vi "Simple Vector Field Histogram.vi"(7 "panic range":T1, 8 "error in (no error)":errorcluster, 9 "distance threshold":dbl, 10 "direction angles":dbl[](array[numeric]), 11 "distances":dbl[](array[numeric])) -> (0 "error out":errorcluster, 1 "histogram":cluster{"Direction":dbl[], dbl[]}[](graph)=[{"Direction"=array[277 elements], [0.5, 0.5, 0.5, 0.5, 0.5, 0.5, 0.5, 0.5, 0.5, 0.5, 0.5, 0.5, 0.5, 0.5, 0.5, 0.5, 0.5, 0.5, 0.5, 0.5, 0.5, 0.5, 0.5, 0.5, 0.5, 0.5, 0.5, 0.5, 0.5, 0.5, 0.5, 0.5, 0.5, 0.5, 0.5, 0.5, 0.5, 0.5, 0.5, 0.5, 0.5, 0.5, 0.5, 0.5, 0.5, 0.5, 0.5, 0.5, 0.5, 0.5, 0.5, 0.5, 0.5, 0.5, 0.5, 0.5, 0.5, 0.5, 0.5, 0.5, 0.5, 0.5, 0.5, 0.5, 0.5, 0.5, 0.5, 0.5, 0.5, 0.5, 0.5, 0.5, 0.5, 0.5, 0.5, 0.5, 0.5, 0.5, 0.5, 0.5, 0.5, 0.5, 0.5, 0.5, 0.5, 0.5, 0.5, 0.5, 0.5, 0.5, 0.5, 0.5, 0.5, 0.5, 0.5, 0.5, 0.5, 0.5, 0.5, 0.5, 0.5, 0.5, 0.5, 0.5, 0.5, 0.5, 0.5, 0.5, 0.5, 0.5, 0.5, 0.5, 0.5, 0.5, 0.5, 0.5, 0.5, 0.5, 0.5, 0.5, 0.5, 0.5, 0.5, 0.5, 0.5, 0.5, 0.5, 0.5, 0.5, 0.5, 0.5, 0.5, 0.5, 0.5, 0.5, 0.5, 0.5, 0.5, 0.5, 0.5, 0.5, 0.5, 0.5, 0.5, 0.5, 0.5, 0.5, 0.5, 0.5, 0.5, 0.5, 0.5, 0.5, 0.5, 0.5, 0.5, 0.5, 0.5, 0.5, 0.5, 0.5, 0.5, 0.5, 0.5, 0.5, 0.5, 0.5, 0.5, 0.5, 0.5, 0.5, 0.5, 0.5, 0.5, 0.5, 0.5, 0.5, 0.5, 0.5, 0.5, 0.5, 0.5, 0.5, 0.5, 0.5, 0.5, 0.5, 0.5, 0.5, 0.5, 0.5, 0.5, 0.5, 0.5, 0.5, 0.5, 0.5, 0.5, 0.5, 0.5, 0.5, 0.5, 0.5, 0.5, 0.5, 0.5, 0.5, 0.5, 0.5, 0.5, 0.5, 0.5, 0.5, 0.5, 0.5, 0.5, 0.5, 0.5, 0.5, 0.5, 0.5, 0.5, 0.5, 0.5, 0.5, 0.5, 0.5, 0.5, 0.5, 0.5, 0.5, 0.5, 0.5, 0.5, 0.5, 0.5, 0.5, 0.5, 0.5, 0.5, 0.5, 0.5, 0.5, 0.5, 0.5, 0.5, 0.5, 0.5, 0.5, 0.5, 0.5, 0.5, 0.5, 0.5, 0.5, 0.5, 0.5, 0.5, 0.5, 0.5, 0.5, 0.5, 0.5, 0.5, 0.5, 0.5, 0.5, 0.5, 0.5, 0.5, 0.5, 0.5, 0.5, 0.5, 0.5, 0.5, 0.5]}, {"Direction"=array[683 elements], [0.0, 1.0, 1.0, 1.0, 1.0, 1.0, 1.0, 1.0, 1.0, 1.0, 1.0, 1.0, 1.0, 1.0, 1.0, 1.0, 1.0, 1.0, 1.0, 1.0, 1.0, 1.0, 1.0, 1.0, 1.0, 1.0, 1.0, 1.0, 1.0, 1.0, 1.0, 1.0, 1.0, 1.0, 1.0, 1.0, 1.0, 1.0, 1.0, 1.0, 1.0, 1.0, 1.0, 1.0, 1.0, 1.0, 1.0, 1.0, 1.0, 1.0, 1.0, 1.0, 1.0, 1.0, 1.0, 1.0, 1.0, 1.0, 1.0, 1.0, 1.0, 1.0, 1.0, 1.0, 1.0, 1.0, 1.0, 1.0, 1.0, 1.0, 1.0, 1.0, 1.0, 1.0, 1.0, 1.0, 1.0, 1.0, 1.0, 1.0, 1.0, 1.0, 1.0, 1.0, 1.0, 1.0, 1.0, 1.0, 1.0, 1.0, 1.0, 1.0, 1.0, 1.0, 1.0, 1.0, 1.0, 1.0, 1.0, 1.0, 1.0, 1.0, 1.0, 1.0, 1.0, 1.0, 1.0, 1.0, 1.0, 1.0, 1.0, 0.0, 0.0, 0.0, 0.0, 0.0, 0.0, 0.0, 0.0, 0.0, 0.0, 0.0, 0.0, 0.0, 0.0, 0.0, 0.0, 0.0, 0.0, 0.0, 0.0, 0.0, 1.0, 1.0, 1.0, 1.0, 1.0, 1.0, 1.0, 1.0, 1.0, 1.0, 1.0, 1.0, 1.0, 1.0, 1.0, 1.0, 1.0, 1.0, 1.0, 1.0, 1.0, 1.0, 1.0, 1.0, 1.0, 1.0, 1.0, 1.0, 1.0, 1.0, 1.0, 1.0, 1.0, 1.0, 1.0, 1.0, 1.0, 1.0, 1.0, 1.0, 1.0, 1.0, 1.0, 1.0, 1.0, 1.0, 1.0, 1.0, 1.0, 1.0, 1.0, 1.0, 1.0, 1.0, 1.0, 1.0, 1.0, 1.0, 1.0, 1.0, 1.0, 1.0, 1.0, 1.0, 1.0, 1.0, 1.0, 1.0, 1.0, 1.0, 1.0, 1.0, 1.0, 1.0, 1.0, 1.0, 1.0, 1.0, 1.0, 1.0, 1.0, 1.0, 1.0, 1.0, 0.0, 0.0, 0.0, 0.0, 0.0, 0.0, 0.0, 0.0, 0.0, 0.0, 0.0, 0.0, 0.0, 0.0, 0.0, 0.0, 0.0, 0.0, 0.0, 0.0, 0.0, 0.0, 0.0, 0.0, 0.0, 0.0, 0.0, 0.0, 0.0, 0.0, 0.0, 0.0, 0.0, 0.0, 0.0, 0.0, 0.0, 0.0, 0.0, 0.0, 0.0, 0.0, 0.0, 0.0, 0.0, 0.0, 0.0, 0.0, 0.0, 0.0, 0.0, 0.0, 0.0, 0.0, 0.0, 0.0, 0.0, 0.0, 0.0, 0.0, 0.0, 0.0, 0.0, 0.0, 0.0, 0.0, 0.0, 0.0, 0.0, 0.0, 0.0, 0.0, 0.0, 0.0, 0.0, 0.0, 0.0, 0.0, 0.0, 0.0, 0.0, 0.0, 0.0, 0.0, 0.0, 0.0, 0.0, 0.0, 0.0, 0.0, 0.0, 0.0, 0.0, 0.0, 0.0, 0.0, 0.0, 0.0, 0.0, 0.0, 0.0, 0.0, 0.0, 0.0, 0.0, 0.0, 0.0, 0.0, 0.0, 0.0, 0.0, 0.0, 0.0, 0.0, 0.0, 0.0, 0.0, 0.0, 0.0, 0.0, 0.0, 0.0, 0.0, 0.0, 0.0, 0.0, 0.0, 0.0, 0.0, 0.0, 0.0, 0.0, 0.0, 0.0, 0.0, 0.0, 0.0, 0.0, 0.0, 0.0, 0.0, 0.0, 0.0, 0.0, 0.0, 0.0, 0.0, 0.0, 0.0, 0.0, 0.0, 0.0, 0.0, 0.0, 0.0, 0.0, 0.0, 0.0, 0.0, 0.0, 0.0, 0.0, 0.0, 0.0, 0.0, 0.0, 0.0, 0.0, 0.0, 0.0, 0.0, 0.0, 0.0, 0.0, 0.0, 0.0, 0.0, 0.0, 0.0, 0.0, 0.0, 0.0, 0.0, 0.0, 0.0, 0.0, 0.0, 0.0, 0.0, 0.0, 0.0, 0.0, 0.0, 0.0, 0.0, 0.0, 0.0, 0.0, 0.0, 0.0, 0.0, 0.0, 0.0, 0.0, 0.0, 0.0, 0.0, 0.0, 0.0, 0.0, 0.0, 0.0, 0.0, 0.0, 0.0, 0.0, 0.0, 0.0, 0.0, 0.0, 0.0, 0.0, 0.0, 0.0, 0.0, 0.0, 0.0, 0.0, 0.0, 0.0, 0.0, 0.0, 0.0, 0.0, 0.0, 0.0, 0.0, 0.0, 0.0, 0.0, 0.0, 0.0, 0.0, 0.0, 0.0, 0.0, 0.0, 0.0, 0.0, 0.0, 0.0, 0.0, 0.0, 0.0, 0.0, 0.0, 0.0, 0.0, 0.0, 0.0, 0.0, 0.0, 0.0, 0.0, 0.0, 0.0, 0.0, 0.0, 0.0, 0.0, 0.0, 0.0, 0.0, 0.0, 0.0, 0.0, 0.0, 1.0, 1.0, 1.0, 1.0, 1.0, 1.0, 1.0, 1.0, 1.0, 1.0, 1.0, 1.0, 1.0, 0.0, 0.0, 0.0, 0.0, 0.0, 0.0, 0.0, 0.0, 0.0, 0.0, 0.0, 0.0, 0.0, 0.0, 0.0, 0.0, 0.0, 0.0, 0.0, 0.0, 0.0, 0.0, 0.0, 0.0, 0.0, 0.0, 0.0, 0.0, 0.0, 0.0, 0.0, 0.0, 0.0, 0.0, 0.0, 0.0, 0.0, 0.0, 0.0, 0.0, 0.0, 0.0, 0.0, 0.0, 0.0, 0.0, 0.0, 0.0, 0.0, 0.0, 0.0, 0.0, 0.0, 0.0, 0.0, 0.0, 0.0, 0.0, 0.0, 0.0, 0.0, 0.0, 0.0, 0.0, 0.0, 1.0, 1.0, 1.0, 1.0, 1.0, 1.0, 1.0, 1.0, 1.0, 1.0, 1.0, 1.0, 1.0, 1.0, 1.0, 1.0, 1.0, 1.0, 1.0, 1.0, 1.0, 1.0, 1.0, 1.0, 1.0, 1.0, 1.0, 1.0, 1.0, 1.0, 1.0, 1.0, 1.0, 1.0, 1.0, 1.0, 1.0, 1.0, 1.0, 1.0, 1.0, 1.0, 1.0, 1.0, 1.0, 1.0, 1.0, 1.0, 1.0, 1.0, 1.0, 1.0, 1.0, 1.0, 1.0, 1.0, 1.0, 1.0, 1.0, 1.0, 1.0, 1.0, 1.0, 1.0, 1.0, 1.0, 1.0, 1.0, 1.0, 1.0, 1.0, 1.0, 1.0, 1.0, 1.0, 1.0, 1.0, 0.0, 0.0, 0.0, 0.0, 0.0, 0.0, 0.0, 0.0, 0.0, 0.0, 0.0, 0.0, 0.0, 0.0, 0.0, 0.0, 0.0, 0.0, 0.0, 0.0, 0.0, 0.0, 0.0, 0.0, 0.0, 0.0, 0.0, 0.0, 0.0, 0.0, 0.0, 0.0, 0.0, 0.0, 0.0]}], 2 "nearest obstacle":T2, 3 "largest gap":T3, 5 "obstacle within panic range":bool)   [LabVIEW 2017, in "NI_Robotics_Simple Vector Field Histogram.lvlib"]
doc: "Identifies obstacles and gaps, or open areas, in the robot environment, which you can use to implement reactionary motion in a robot vehicle."
uses:
  <vilib>/robotics/Obstacle Avoidance/Simple Vector Field Histogram/NI_Robotics_Simple Vector Field Histogram.lvlib
  <vilib>/robotics/Obstacle Avoidance/Simple Vector Field Histogram/Gap Description.ctl
  <vilib>/robotics/Obstacle Avoidance/Simple Vector Field Histogram/Obstacle Description.ctl
  <vilib>/robotics/Obstacle Avoidance/Simple Vector Field Histogram/Panic Range.ctl
  <vilib>/robotics/Obstacle Avoidance/Simple Vector Field Histogram/Simple VFH Score.vi
  <vilib>/gmath/statdist.llb/Continuous PDF.vi
  <vilib>/gmath/statdist.llb/Normal PDF.vi
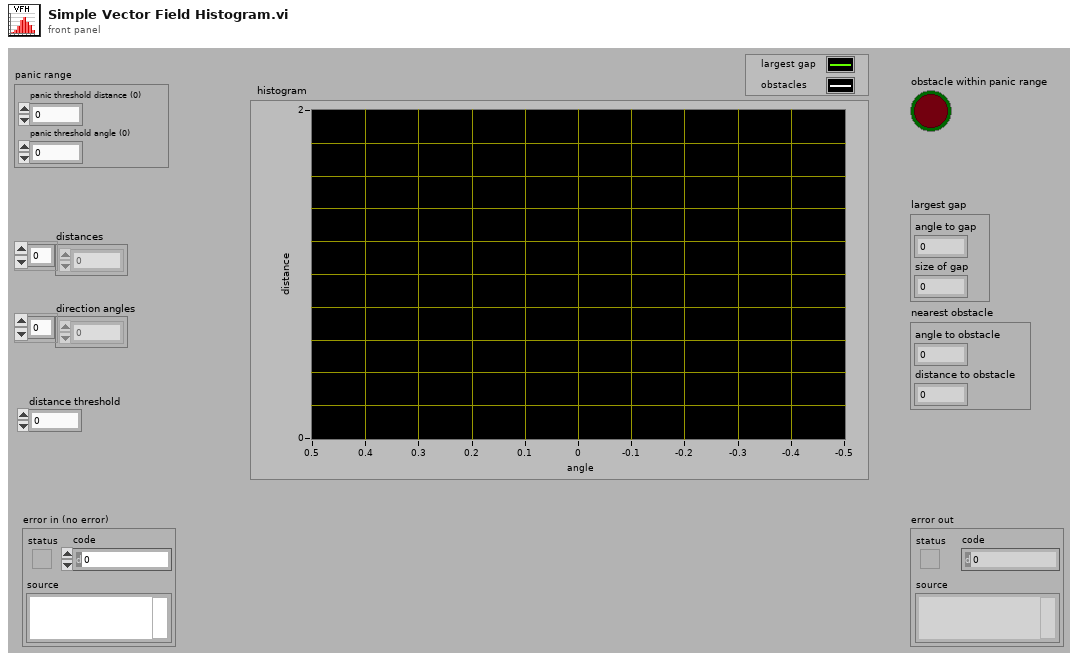
[diagram p1: front panel]
types:
  T1 = typedef "NI_Robotics_Simple Vector Field Histogram.lvlib/Panic Range.ctl" = cluster{"panic threshold distance (0)":dbl, "panic threshold angle (0)":dbl}
  T2 = typedef "NI_Robotics_Simple Vector Field Histogram.lvlib/Obstacle Description.ctl" = cluster{"angle to obstacle":dbl, "distance to obstacle":dbl}
  T3 = typedef "NI_Robotics_Simple Vector Field Histogram.lvlib/Gap Description.ctl" = cluster{"angle to gap":dbl, "size of gap":dbl}
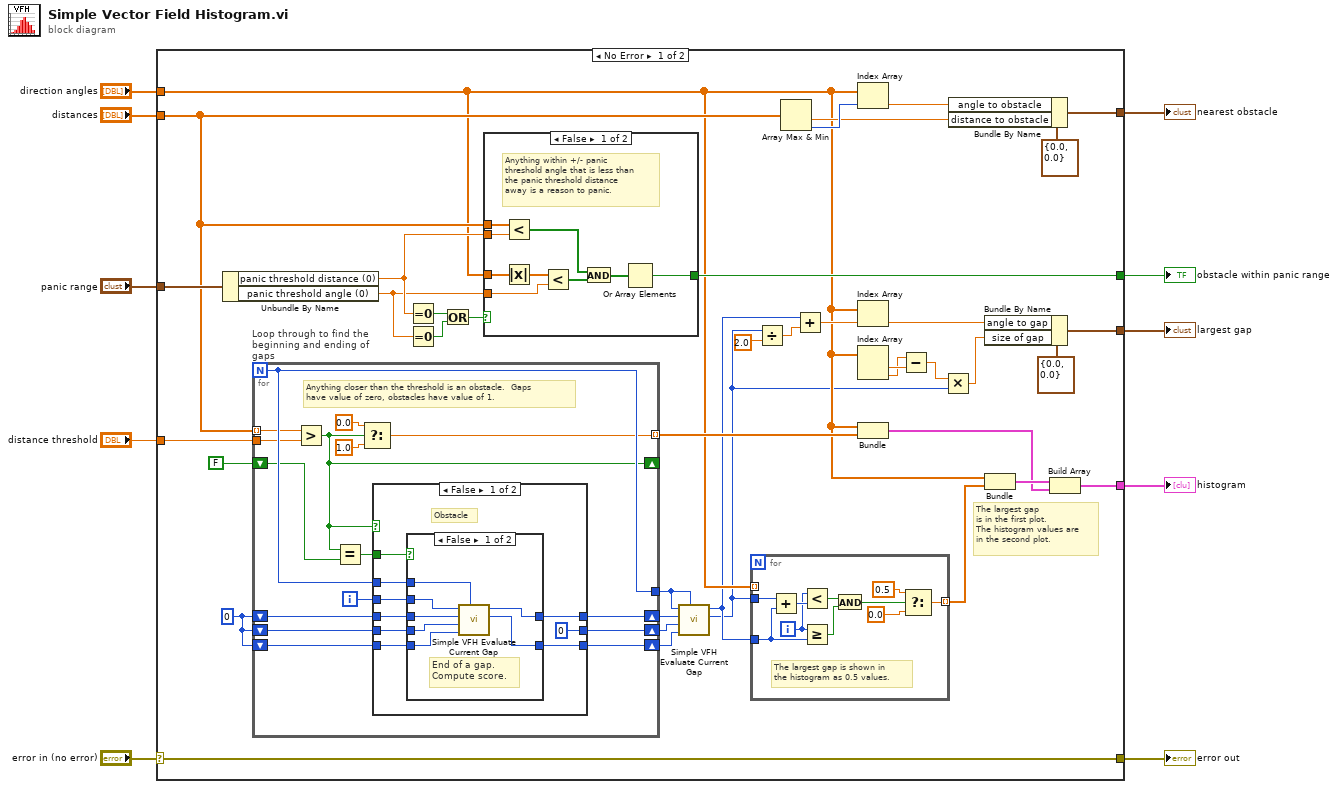
[diagram p0: block diagram]
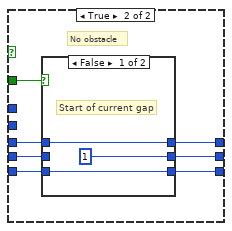
[diagram p4: hidden frame]
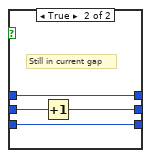
[diagram p5: hidden frame]
diagram:
  n1 = case shown="No Error" "error in (no error)" {
    selector: "error in (no error)" -> [w24 w117]
    tunnel: [w44 _] -> w10
    tunnel: [w35 _] -> w9
    tunnel: "distance threshold" -> [w34 _]
    tunnel: "distances" -> [w23 _]
    tunnel: "direction angles" -> [w14 _]
    tunnel: "panic range" -> [w30 _]
    tunnel: [w24 w117] -> w3
    tunnel: [w21 _] -> w2
    tunnel: [w16 _] -> w1
    frame No Error {
      w42 = 0
      # "The largest gap\nis in the first plot.\nThe histogram values are\nin the second plot."
      n2 = Unbundle By Name(w30) -> ("panic threshold distance (0)"=w29:dbl, "panic threshold angle (0)"=w28:dbl)
      n3 = for "Loop through to find the beginning and ending of gaps" {
        N -> [w77]
        shift-right: [w81] -> w48
        shift-left: w42 -> [w82]
        shift-right: [w83] -> w46
        shift-left: w42 -> [w84]
        shift-right: [w78] -> w47
        shift-left: w42 -> [w80]
        tunnel: [w77] -> w49
        tunnel: w34 -> [w74]
        tunnel: w23 -> [w75] mode=indexing
        tunnel: [w71] -> w33 mode=indexing
        shift-right: [w69] -> _
        shift-left: FALSE -> [w70]
        i -> [w79]
        # "Anything closer than the threshold is an obstacle.  Gaps\nhave value of zero, obstacles have value of 1."
        n4 = Greater?(x=w75, y=w74) -> (0:w69:bool)
        n5 = Equal?(x=w69, y=w70) -> (x = y?=w76:bool)
        n6 = Select(t=0.0, s=w69, f=1.0) -> (s? t:f=w71:dbl)
        n7 = case shown="False" w69 {
          tunnel: w84 -> [w92 w109]
          tunnel: [0 w108] -> w83
          tunnel: w82 -> [w90 w107]
          tunnel: [w91 w106] -> w81
          tunnel: w80 -> [w89 w105]
          tunnel: [w87 w104] -> w78
          tunnel: w79 -> [w88 _]
          tunnel: w77 -> [w86 _]
          tunnel: w76 -> [w85 w103]
          frame False {
            # "Obstacle"
            n8 = case shown="False" w85 {
              tunnel: w92 -> [w97 _]
              tunnel: w90 -> [w100 w101]
              tunnel: [w94 w101] -> w91
              tunnel: w89 -> [w99 w102]
              tunnel: w88 -> [w98 _]
              tunnel: [w95 w102] -> w87
              tunnel: w86 -> [w96 _]
              frame False {
                # "End of a gap.  Compute score."
                n9 = call <vilib>:"Simple VFH Evaluate Current Gap.vi"("total sample size"=w96, "size of best gap so far"=w100, "size of gap"=w97, "offset of best gap so far"=w99, "offset of end of gap"=w98) -> ("size of best gap so far"=w94:i32, "offset of best gap so far"=w95:i32)  [unwired: 1 in, 2 out]
              }
              frame True {
                # "Still an obstacle"
              }
            }
          }
          frame True {
            # "No obstacle"
            n10 = case shown="False" w103 {
              tunnel: w109 -> [_ w116]
              tunnel: [1 w115] -> w108
              tunnel: w107 -> [w110 w114]
              tunnel: [w110 w114] -> w106
              tunnel: w105 -> [w111 w113]
              tunnel: [w111 w113] -> w104
              frame False {
                # "Start of current gap"
              }
              frame True {
                # "Still in current gap"
                n11 = Increment(x=w116) -> (x+1=w115:i32)
              }
            }
          }
        }
      }
      n12 = Equal To 0?(x=w29) -> (x = 0?=w27:bool)
      n13 = Equal To 0?(x=w28) -> (x = 0?=w26:bool)
      n14 = Or(x=w27, y=w26) -> (x .or. y?=w25:bool)
      n15 = case shown="False" w25 {
        tunnel: [w67 _] -> w35
        tunnel: w23 -> [w66 _]
        tunnel: w14 -> [w65 _]
        tunnel: w29 -> [w61 _]
        tunnel: w28 -> [w60 _]
        frame False {
          # "Anything within +/- panic\nthreshold angle that is less than\nthe panic threshold distance\naway is a reason to panic."
          n16 = Less?(x=w66, y=w61) -> (x < y?=w62:bool[])
          n17 = Absolute Value(x=w65) -> (abs(x)=w64:dbl[])
          n18 = Less?(x=w64, y=w60) -> (x < y?=w63:bool[])
          n19 = And(x=w62, y=w63) -> (x .and. y?=w68:bool[])
          n20 = Or Array Elements(Boolean array=w68) -> (logical OR=w67:bool)
        }
        frame True {
          # "Do nothing if the panic threshold distance or angle is zero."
        }
      }
      n21 = call <vilib>:"Simple VFH Evaluate Current Gap.vi"("total sample size"=w49, "size of best gap so far"=w48, "size of gap"=w46, "offset of best gap so far"=w47, "offset of end of gap"=w49) -> ("size of best gap so far"=w12:i32, "offset of best gap so far"=w13:i32)  [unwired: 1 in, 2 out]
      n22 = for {
        tunnel: w14 -> [_] mode=indexing
        tunnel: w13 -> [w59]
        tunnel: w12 -> [w58]
        tunnel: [w50] -> w11 mode=indexing
        i -> [w53]
        # "The largest gap is shown in\nthe histogram as 0.5 values."
        n23 = Add(x=w58, y=w59) -> (x+y=w54:i32)
        n24 = Less?(x=w53, y=w54) -> (x < y?=w57:bool)
        n25 = Greater Or Equal?(x=w53, y=w59) -> (x >= y?=w56:bool)
        n26 = And(x=w57, y=w56) -> (x .and. y?=w55:bool)
        n27 = Select(t=0.5, s=w55, f=0.0) -> (s? t:f=w50:dbl)
      }
      n28 = Divide(x=w12, y=2.0) -> (x/y=w40:dbl)
      n29 = Array Max & Min(array=w23) -> (min value=w17:dbl, min index (indices)=w31:i32)  [unwired: 2 out]
      n30 = Add(x=w13, y=w40) -> (x+y=w39:dbl)
      n31 = Index Array(array=w14, index=w31) -> (element=w18:dbl)
      n32 = Index Array(array=w14, index=w39) -> (element=w20:dbl)
      n33 = Index Array(array=w14) -> (element #1=w38:dbl, element #2=w37:dbl)  [unwired: 2 in]
      n34 = Bundle("direction angles"=w14, w33) -> (w43:cluster{"direction angles":dbl[], dbl[]})  [unwired: 1 out]
      n35 = Subtract(x=w37, y=w38) -> (x-y=w36:dbl)
      n36 = Multiply(x=w36, y=w12) -> (x*y=w15:dbl)
      n37 = Bundle By Name(cluster=T2 {"angle to obstacle"=0.0, "distance to obstacle"=0.0} ("nearest obstacle"), "angle to obstacle"=w18, "distance to obstacle"=w17) -> (w16:T2)
      n38 = Bundle By Name(cluster=T3 {"angle to gap"=0.0, "size of gap"=0.0} ("largest gap"), "angle to gap"=w20, "size of gap"=w15) -> (w21:T3)
      n39 = Bundle("direction angles"=w14, w11) -> (w45:cluster{"direction angles":dbl[], dbl[]})  [unwired: 1 out]
      n40 = Build Array(w45, w43) -> (w44:cluster{"direction angles":dbl[], dbl[]}[])
    }
    frame Error {
    }
  }
  "histogram" <- w10
  "obstacle within panic range" <- w9
  "largest gap" <- w2
  "nearest obstacle" <- w1
  "error out" <- w3
